vi "Test Case Skip and Pass Gives Pass Result.vi"(8 "error in (no error)":errorcluster, 11 "Test Test Case Result In":refnum<class "Test Case Result Test.lvclass">) -> (0 "error out":errorcluster, 3 "Test Test Case Result Out":refnum<class "Test Case Result Test.lvclass">)   [LabVIEW 2020, in "LUnit Tests.lvlib" / "Test Case Result Test.lvclass"]
uses:
  Test Case Result Test.lvclass
  C:/Program Files (x86)/National Instruments/LabVIEW 2020/vi.lib/Astemes/LUnit/Test Case.lvclass
  source/Framework/Result Types/Assertion Result/Public/TypeDefs/Status.ctl
  Skip and Pass Test Case/Skip and Pass Test Case.lvclass
  C:/Git/astemes-lunit/source/Framework/Test Case/LUnit Test Case.lvclass
  <vilib>/Astemes/LUnit/Test Case.lvclass/Test Case.ctl
  source/Framework/Result Types/Case Result/Private/Merge Status.vi
  <vilib>/Astemes/LUnit/Palette/Fail.vi
  <vilib>/Astemes/LUnit/Palette/Pass.vi
  <vilib>/Astemes/LUnit/Set Assertion Type.vi
  <vilib>/Astemes/LUnit/Add test result.vi
  <vilib>/Astemes/LUnit/LUnit Record Assertion Result.vi
  <vilib>/Astemes/LUnit/LUnit Aggregate Assertion Results.vi
  <vilib>/Astemes/LUnit/Method Result/LUnit Merge Status.vi
  <vilib>/Astemes/LUnit/LUnit Concatenate result strings.vi
  source/Framework/Result Types/Case Result/Test Case Result.lvlib
  source/Framework/Result Types/Assertion Result/Assertion Result.lvlib
  <vilib>/Astemes/LUnit/Test Case.lvclass
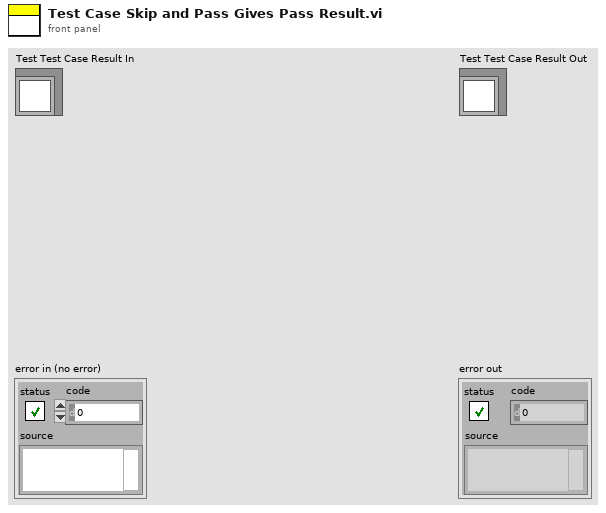
[diagram p1: front panel]
types:
  T1 = typedef "Assertion Result.lvlib/Status.ctl" = enum16{"Pass", "Fail", "Error", "Skipped", "Setup Error", "Broken", "Teardown Error"}
  T2 = typedef "Test Case Result.lvlib/Test Case Result.ctl" = map{string, T3}
  T3 = typedef "Method Result.lvlib/Method Result.ctl" = cluster{"Test Case":string, "Test Method Name":string, "Status":T1, "Assertion Results":T4[], "Execution time":dbl, "Result String":string}
  T4 = typedef "Assertion Result.lvlib/Assertion Result.ctl" = cluster{"Status":T1, "Message":string, "Description":string, "Assertion Type":T5}
  T5 = typedef "Assertion Result.lvlib/Assertion Type.ctl" = enum16{"None", "Pass", "Fail", "Skip", "Pass if Equal", "Fail if Equal", "Pass if Error", "Fail if Error", "Pass if", "Fail if"}
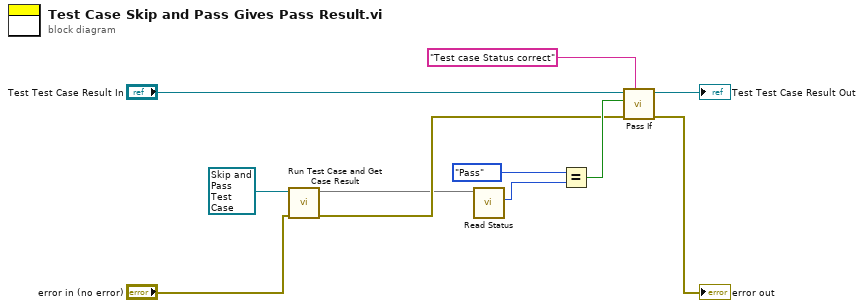
[diagram p0: block diagram]
diagram:
  n1 = call "Run Test Case and Get Case Result.vi"("error in (no error)"="error in (no error)", "Error First Test Case in"=refnum<class "Skip and Pass Test Case.lvclass"> refnum ("Skip and Pass Test Case.lvclass")) -> ("error out"=w4:errorcluster, "Test Case Result out"=w3:T2)  [unwired: 8 in]
  n2 = call "Read Status.vi"("Test Case Result In"=w3) -> ("Status"=w7:T1)  [unwired: 8 in, 2 out]
  n3 = Equal?(x=Status."Pass" ("Status"), y=w7) -> (x = y?=w6:bool)
  n4 = call <vilib>:"Pass If.vi"("Description"="Test case Status correct", "error in (no error)"=w4, "Pass?"=w6, "LUnit Test Case In"="Test Test Case Result In") -> ("error out"=→"error out":errorcluster, "LUnit Test Case Out"=→"Test Test Case Result Out":refnum<class "Test Case Result Test.lvclass">)  [unwired: 6 in]
